vi "Test_SendRoundTripMessage_ReceiveReply_NoError.vi"(8 "error in (no error)":errorcluster, 11 "TestCase in":refnum<class "TestRoundTripMessage.lvclass">) -> (0 "error out":errorcluster, 3 "TestCase out":refnum<class "TestRoundTripMessage.lvclass">)   [LabVIEW 2017, in "TestRoundTripMessage.lvclass"]
uses:
  TestRoundTripMessage.lvclass
  <vilib>/ActorFramework/Actor/Actor.lvclass
  <vilib>/ActorFramework/Message Queue/Message Queue.lvclass/Message Queue.ctl
  <vilib>/ActorFramework/Message Dequeuer/Message Dequeuer.lvclass/Message Dequeuer.ctl
  <vilib>/ActorFramework/Message Enqueuer/Message Enqueuer.lvclass/Message Enqueuer.ctl
  <vilib>/ActorFramework/Message Enqueuer/Enqueue.vi
  <vilib>/ActorFramework/Stop Msg/Stop Msg.lvclass
  C:/Program Files (x86)/National Instruments/LabVIEW 2017/vi.lib/ActorFramework/Message/Message.lvclass
  Doubles/ImmediateReturnRoundTripMessage/ImmediateReturnRoundTripMessage.lvclass
  <vilib>/ActorFramework/Message Priority Queue/Priority Enqueue.vi
  <vilib>/ActorFramework/Message Priority Queue/Priority Dequeue.vi
  <vilib>/ActorFramework/Message Queue/Message Queue.lvclass
  <vilib>/ActorFramework/Message Dequeuer/Message Dequeuer.lvclass
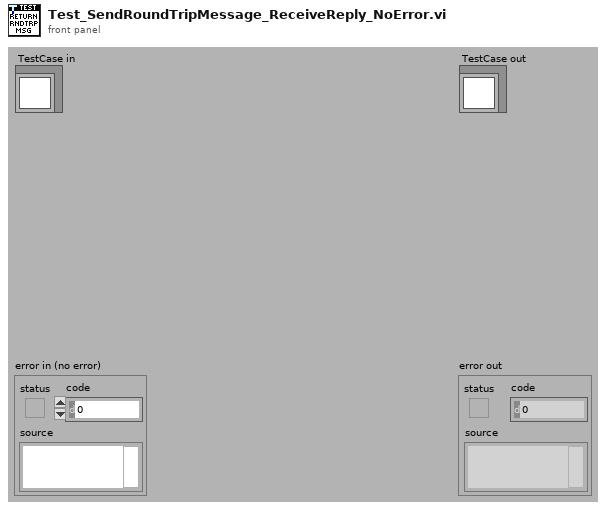
[diagram p1: front panel]
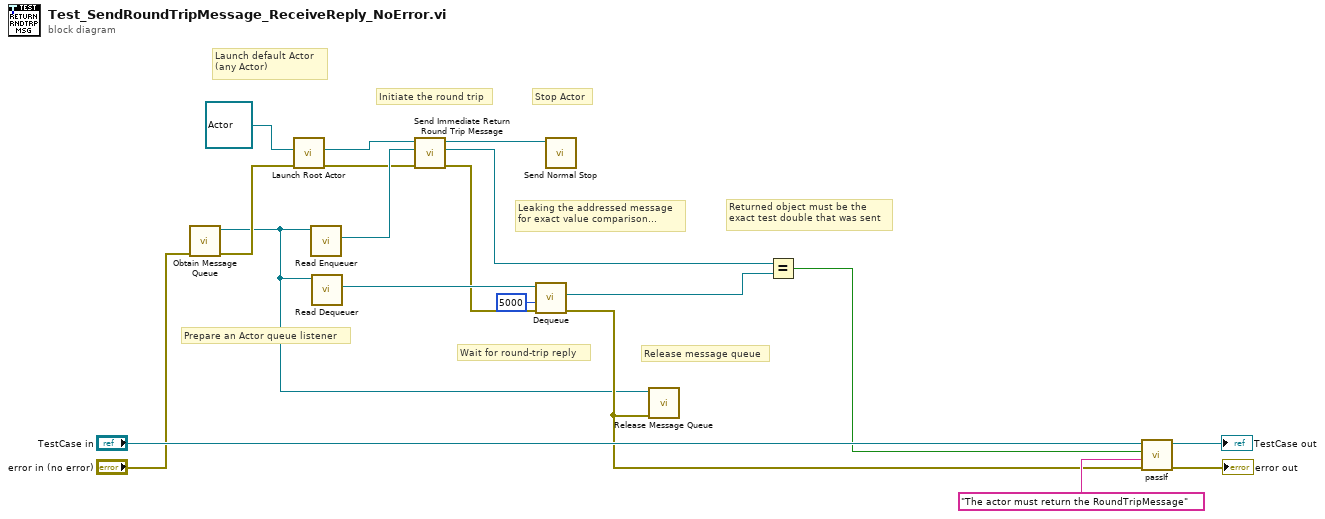
[diagram p0: block diagram]
diagram:
  # "Release message queue"
  # "Leaking the addressed message\nfor exact value comparison..."
  # "Returned object must be the\nexact test double that was sent"
  # "Prepare an Actor queue listener"
  # "Wait for round-trip reply"
  # "Initiate the round trip"
  # "Stop Actor"
  # "Launch default Actor\n(any Actor)"
  n1 = call <vilib>:"Obtain Message Queue.vi"("error in (no error)"="error in (no error)") -> ("error out"=w11:errorcluster, "Message Queue"=w1:refnum<class "Message Queue.lvclass">)  [unwired: 9 in]
  n2 = call <vilib>:"Launch Root Actor.vi"("error in (no error)"=w11, "Actor"=refnum<class "Actor.lvclass"> refnum) -> ("error out"=w10:errorcluster, "Actor's Enqueuer"=w9:refnum<class "Message Enqueuer.lvclass">)  [unwired: 8 in]
  n3 = call <vilib>:"Read Enqueuer.vi"("Message Queue"=w1) -> ("Message Enqueuer"=w15:refnum<class "Message Enqueuer.lvclass">)  [unwired: 10 in]
  n4 = call <vilib>:"Read Dequeuer.vi"("Message Queue"=w1) -> ("Message Dequeuer"=w14:refnum<class "Message Dequeuer.lvclass">)  [unwired: 10 in]
  n5 = call "Send Immediate Return Round Trip Message.vi"("error in (no error)"=w10, "Return Enqueuer (Self)"=w15, "Message Enqueuer (Remote Actor)"=w9) -> ("error out"=w7:errorcluster, "Leak The Round-Trip Message For Test"=w3:refnum<class "ImmediateReturnRoundTripMessage.lvclass">, "Message Enqueuer out"=w8:refnum<class "Message Enqueuer.lvclass">)  [unwired: 6 in]
  n6 = call <vilib>:"Dequeue.vi"("error in (no error)"=w7, "timeout in ms (-1)"=5000, "Message Dequeuer in"=w14) -> ("error out"=w2:errorcluster, "Message"=w6:refnum<class "Message.lvclass">)  [unwired: 4 in, 3 out]
  n7 = call <vilib>:"Send Normal Stop.vi"("Message Enqueuer"=w8) -> ()  [unwired: 10 in, 1 out]
  n8 = call <vilib>:"Release Message Queue.vi"("error in (no error)"=w2, "Message Queue"=w1) -> ()  [unwired: 8 in, 2 out]
  n9 = Equal?(x=w3, y=w6) -> (x = y?=w5:bool)
  n10 = call-dynamic "passIf.vi"("error in (no error)"=w2, "message (\"\")"="The actor must return the RoundTripMessage" ("message (\"\")"), "pass"=w5, "TestCase in"="TestCase in") -> ("error out"=→"error out":errorcluster, "TestCase out"=→"TestCase out":refnum<class "TestRoundTripMessage.lvclass">)  [unwired: 6 in]
